vi "niRFSysCalReader Core.vi"(4 "Enable Interpolation?":bool=TRUE, 6 "CalData":dbl[](array[numeric]), 7 "Frequency (Hz)":dbl, 8 "error in":errorcluster, 9 "niRFSysCalReader State":T1, 10 "Power (dBm)":dbl, 11 "niRFSysCalReader Handle":T2) -> (0 "error out":errorcluster, 2 "CalData Out":dbl[](array[numeric]), 3 "niRFSysCalReader Handle out":T2)   [LabVIEW 2018, in "niRFSysCalReader.lvlib"]
doc: "Core component of the niRFSysCalReader library."
uses:
  niRFSysCalReader.lvlib
  INCLUDES/niRFSysCalReader Handle.ctl
  INCLUDES/niRFSysCalReader Core States.ctl
  <vilib>/Utility/error.llb/Error Cluster From Error Code.vi
  <vilib>/ErrorRing/Error Ring.xnode
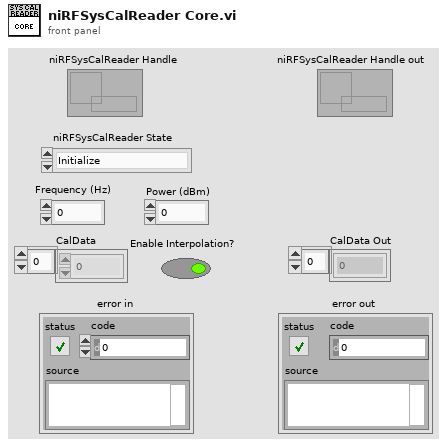
[diagram p1: front panel]
types:
  T1 = typedef "niRFSysCalReader.lvlib/niRFSysCalReader Core States.ctl" = enum16{"Initialize", "Interpolator State", "Add CalData", "Get CalData", "Remove Pathloss", "Close"}
  T2 = typedef "niRFSysCalReader.lvlib/niRFSysCalReader Handle.ctl" = refnum<data-value>
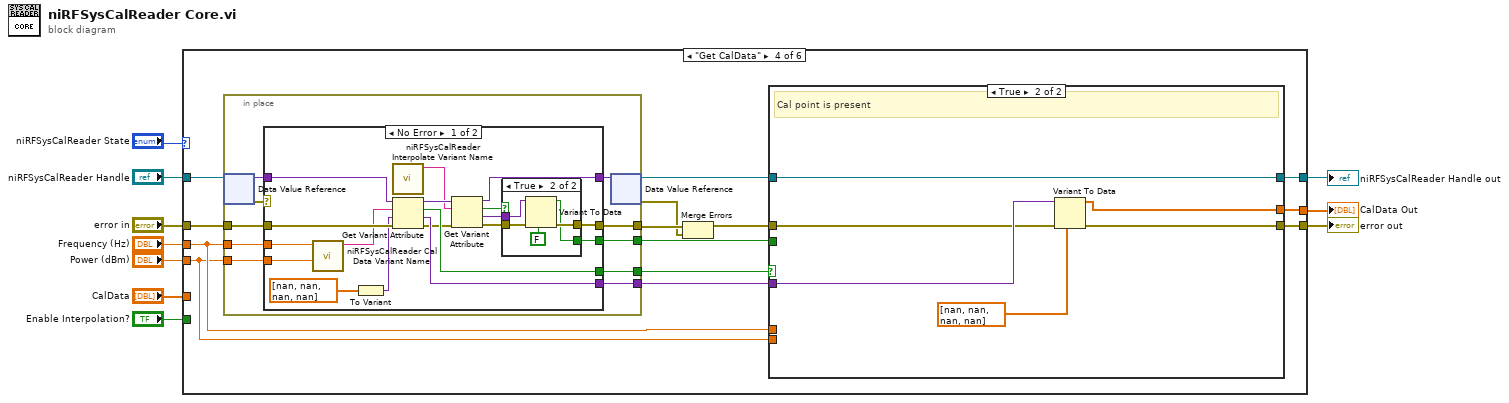
[diagram p0: block diagram]
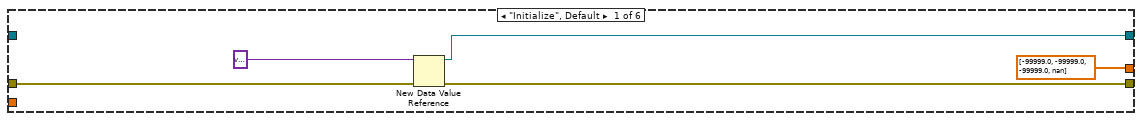
[diagram p2: hidden frame]
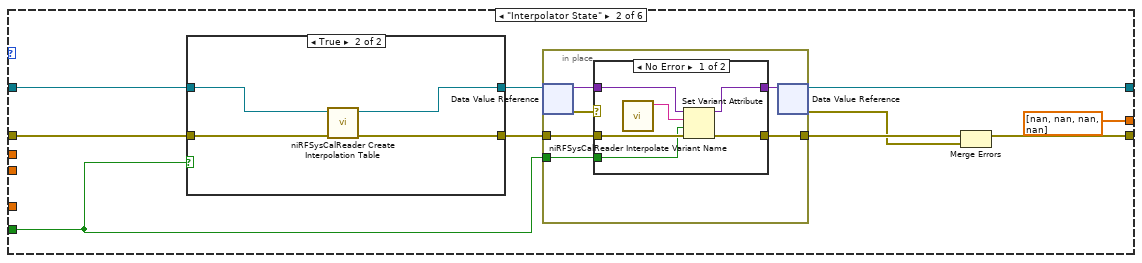
[diagram p3: hidden frame]
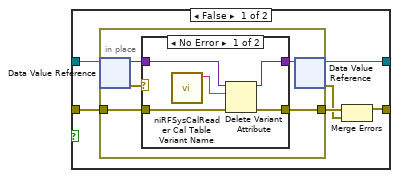
[diagram p4: hidden frame]
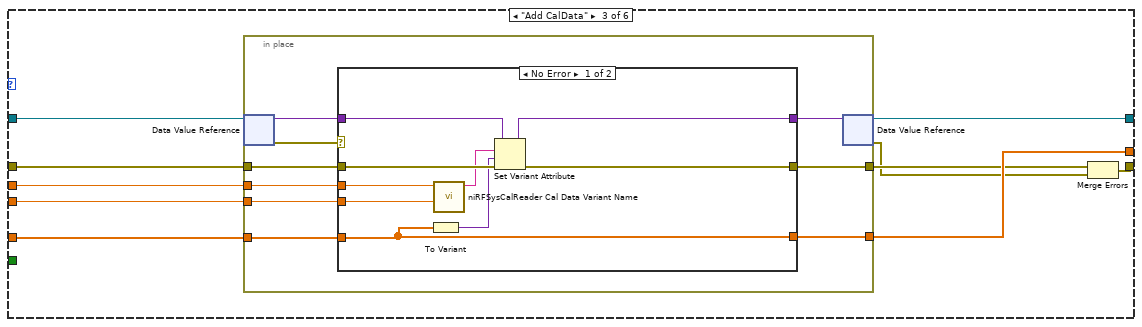
[diagram p7: hidden frame]
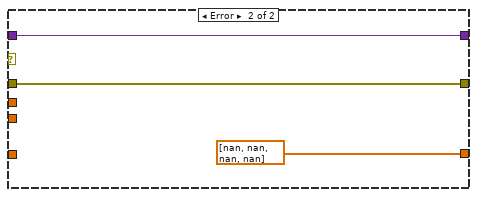
[diagram p8: hidden frame]
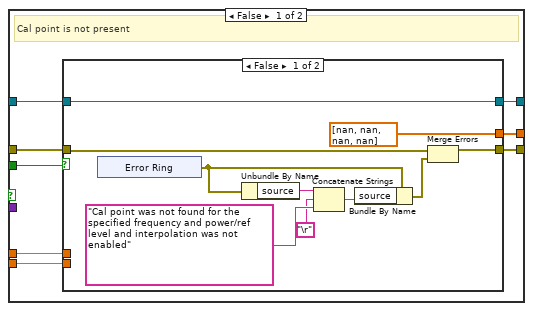
[diagram p9: hidden frame]
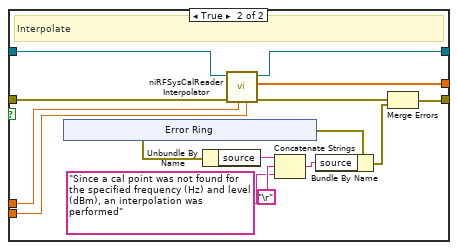
[diagram p10: hidden frame]
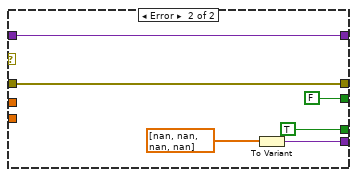
[diagram p12: hidden frame]
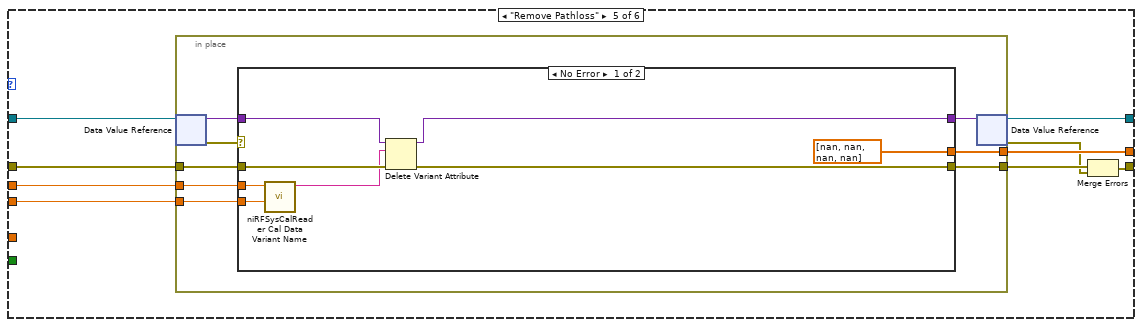
[diagram p13: hidden frame]
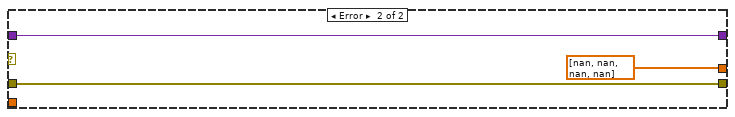
[diagram p14: hidden frame]
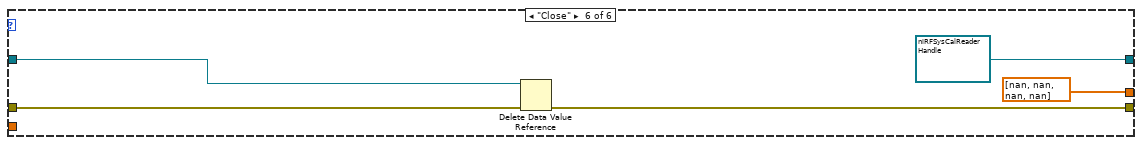
[diagram p15: hidden frame]
diagram:
  n1 = case shown="\"Get CalData\"" "niRFSysCalReader State" {
    tunnel: [w14 w25 w69 w97 w200 T2 refnum ("Cal Storage Handle in")] -> w5
    tunnel: [w13 w24 w68 w100 w199 w224] -> w4
    tunnel: "error in" -> [w12 w21 w70 w105 w201 w225]
    tunnel: "niRFSysCalReader Handle" -> [_ w23 w71 w106 w202 w226]
    tunnel: "Frequency (Hz)" -> [_ _ w67 w96 w198 _]
    tunnel: "Power (dBm)" -> [_ _ w66 w95 w197 _]
    tunnel: [dbl[] [-99999.0, -99999.0, -99999.0, nan] dbl[] [nan, nan, nan, nan] w65 w99 w196 dbl[] [nan, nan, nan, nan]] -> w1
    tunnel: "Enable Interpolation?" -> [_ w17 _ _ _ _]
    tunnel: "CalData" -> [_ _ w62 _ _ _]
    frame "Initialize", Default {
      n2 = New Data Value Reference(data value=variant, error in=w12) -> (data value reference=w14:refnum<data-value>, error out=w13:errorcluster)
    }
    frame "Interpolator State" {
      n3 = case shown="True" w17 {
        tunnel: w23 -> [w31 w47]
        tunnel: [w30 w46] -> w22
        tunnel: w21 -> [w29 w45]
        tunnel: [w28 w44] -> w20
        frame False {
          n4 = in-place {
            in-place-border: w29 -> [w34]
            in-place-border: [w33] -> w27
            n5 = in-place-dvr #1(w31) -> (w36:variant, w32:errorcluster)
            n6 = case shown="No Error" w32 {
              tunnel: w36 -> [w41 w43]
              tunnel: [w40 w43] -> w35
              tunnel: w34 -> [w39 w42]
              tunnel: [w38 w42] -> w33
              frame No Error {
                n7 = call "niRFSysCalReader Cal Table Variant Name.vi"() -> ("Calibration Table Name"=w37:string)  [unwired: 11 in]
                n8 = Delete Variant Attribute(4:w39, 6:w37, 7:w41) -> (0:w38:errorcluster, 3:w40:variant)  [unwired: 1 out]
              }
              frame Error {
              }
            }
            n9 = in-place-dvr #1(w35) -> (w30:T2, w26:errorcluster)
          }
          n10 = Merge Errors(w27, w26) -> (w28:errorcluster)
        }
        frame True {
          n11 = call "niRFSysCalReader Create Interpolation Table.vi"("error in"=w45, "niRFSysCalReader Handle"=w47) -> ("error out"=w44:errorcluster, "niRFSysCalReader Handle out"=w46:T2)  [unwired: 7 in, 1 out]
        }
      }
      n12 = in-place {
        in-place-border: [w52] -> w19
        in-place-border: w20 -> [w50]
        in-place-border: w17 -> [w48]
        n13 = in-place-dvr #2(w22) -> (w53:variant, w49:errorcluster)
        n14 = case shown="No Error" w49 {
          tunnel: w53 -> [w59 w61]
          tunnel: [w57 w60] -> w52
          tunnel: [w56 w61] -> w51
          tunnel: w50 -> [w55 w60]
          tunnel: w48 -> [w54 _]
          frame No Error {
            n15 = call "niRFSysCalReader Interpolate Variant Name.vi"() -> ("Interpolation State Name"=w58:string)  [unwired: 11 in]
            n16 = Set Variant Attribute(Variant=w59, name=w58, value=w54, error in=w55) -> (Variant out=w56:variant, error out=w57:errorcluster)  [unwired: 1 out]
          }
          frame Error {
          }
        }
        n17 = in-place-dvr #2(w51) -> (w25:T2, w18:errorcluster)
      }
      n18 = Merge Errors(w19, w18) -> (w24:errorcluster)
    }
    frame "Add CalData" {
      n19 = in-place {
        in-place-border: w70 -> [w79]
        in-place-border: [w76] -> w64
        in-place-border: w67 -> [w75]
        in-place-border: w66 -> [w74]
        in-place-border: [w73] -> w65
        in-place-border: w62 -> [w72]
        n20 = in-place-dvr #3(w71) -> (w78:variant, w80:errorcluster)
        n21 = case shown="No Error" w80 {
          tunnel: w79 -> [w89 w91]
          tunnel: w78 -> [w84 w92]
          tunnel: [w83 w92] -> w77
          tunnel: [w88 w91] -> w76
          tunnel: w75 -> [w87 _]
          tunnel: w74 -> [w86 _]
          tunnel: w72 -> [w81 _]
          tunnel: [w81 dbl[] [nan, nan, nan, nan]] -> w73
          frame No Error {
            n22 = To Variant(anything=w81) -> (Variant=w82:variant)
            n23 = call "niRFSysCalReader Cal Data Variant Name.vi"("Power (dBm)"=w86, "Frequency (Hz)"=w87) -> ("Calibration Data Name"=w85:string)  [unwired: 9 in]
            n24 = Set Variant Attribute(Variant=w84, name=w85, value=w82, error in=w89) -> (Variant out=w83:variant, error out=w88:errorcluster)  [unwired: 1 out]
          }
          frame Error {
          }
        }
        n25 = in-place-dvr #3(w77) -> (w69:T2, w63:errorcluster)
      }
      n26 = Merge Errors(w64, w63) -> (w68:errorcluster)
    }
    frame "Get CalData" {
      n27 = in-place {
        in-place-border: w105 -> [w161]
        in-place-border: [w158] -> w104
        in-place-border: w96 -> [w157]
        in-place-border: w95 -> [w156]
        in-place-border: [w155] -> w93
        in-place-border: [w154] -> w102
        in-place-border: [w153] -> w94
        n28 = in-place-dvr #4(w106) -> (w160:variant, w162:errorcluster)
        n29 = case shown="No Error" w162 {
          tunnel: w161 -> [w180 w192]
          tunnel: w160 -> [w178 w193]
          tunnel: [w170 w193] -> w159
          tunnel: [w168 w192] -> w158
          tunnel: w157 -> [w176 _]
          tunnel: w156 -> [w175 _]
          tunnel: [w174 w188] -> w154
          tunnel: [w173 TRUE] -> w155
          tunnel: [w165 FALSE] -> w153
          frame No Error {
            n30 = call "niRFSysCalReader Cal Data Variant Name.vi"("Power (dBm)"=w175, "Frequency (Hz)"=w176) -> ("Calibration Data Name"=w179:string)  [unwired: 9 in]
            n31 = To Variant(anything=dbl[] [nan, nan, nan, nan]) -> (Variant=w177:variant)
            n32 = call "niRFSysCalReader Interpolate Variant Name.vi"() -> ("Interpolation State Name"=w164:string)  [unwired: 11 in]
            n33 = Get Variant Attribute(Variant=w178, name=w179, default value (empty Variant)=w177, error in=w180) -> (duplicate Variant=w171:variant, found=w173:bool, value=w174:variant, error out=w172:errorcluster)
            n34 = Get Variant Attribute(Variant=w171, name=w164, error in=w172) -> (duplicate Variant=w170:variant, found=w166:bool, value=w167:variant, error out=w169:errorcluster)  [unwired: 1 in]
            n35 = case shown="True" w166 {
              selector: w166 -> [w182 _]
              tunnel: w169 -> [w181 w187]
              tunnel: [w181 w186] -> w168
              tunnel: w167 -> [_ w185]
              tunnel: [w182 w183] -> w165
              frame False {
              }
              frame True {
                n36 = Variant To Data(error in=w187, type=FALSE, Variant=w185) -> (data=w183:bool, error out=w186:errorcluster)
              }
            }
          }
          frame Error {
            n37 = To Variant(anything=dbl[] [nan, nan, nan, nan]) -> (Variant=w188:variant)
          }
        }
        n38 = in-place-dvr #4(w159) -> (w98:T2, w103:errorcluster)
      }
      n39 = Merge Errors(w104, w103) -> (w101:errorcluster)
      n40 = case shown="True" w93 {
        tunnel: [w114 w152] -> w100
        tunnel: [w113 w151] -> w99
        tunnel: w102 -> [_ w150]
        tunnel: w101 -> [w112 w149]
        tunnel: w98 -> [w111 w148]
        tunnel: [w110 w148] -> w97
        tunnel: w94 -> [w109 _]
        tunnel: w96 -> [w108 _]
        tunnel: w95 -> [w107 _]
        frame False {
          # "Cal point is not present"
          n41 = case shown="False" w109 {
            tunnel: [w122 w134] -> w114
            tunnel: [dbl[] [nan, nan, nan, nan] w142] -> w113
            tunnel: w112 -> [w123 w141]
            tunnel: w111 -> [w124 w140]
            tunnel: [w124 w139] -> w110
            tunnel: w108 -> [_ w130]
            tunnel: w107 -> [_ w129]
            frame False {
              n42 = xnode "Error Ring"() -> ("error out"=w121:errorcluster)
              n43 = Unbundle By Name(w121) -> ("source"=w118:string)
              n44 = Concatenate Strings(w118, "\r", "Cal point was not found for the specified frequency and power/ref level and interpolation was not enabled" ("error message (\"\")")) -> (w117:string)
              n45 = Bundle By Name(cluster=w121, "source"=w117) -> (w116:errorcluster)
              n46 = Merge Errors(w123, w116) -> (w122:errorcluster)
            }
            frame True {
              # "Interpolate"
              n47 = xnode "Error Ring"() -> ("error out"=w131:errorcluster)
              n48 = Unbundle By Name(w131) -> ("source"=w137:string)
              n49 = call "niRFSysCalReader Interpolator.vi"("Power (dBm)"=w129, "Frequency (Hz)"=w130, "error in"=w141, "niRFSysCalReader Handle"=w140) -> ("error out"=w133:errorcluster, "Interpolated Pathloss (dB)"=w142:dbl[], "niRFSysCalReader Handle out"=w139:T2)  [unwired: 5 in]
              n50 = Concatenate Strings(w137, "\r", "Since a cal point was not found for the specified frequency (Hz) and level (dBm), an interpolation was performed" ("error message (\"\")")) -> (w138:string)
              n51 = Bundle By Name(cluster=w131, "source"=w138) -> (w132:errorcluster)
              n52 = Merge Errors(w133, w132) -> (w134:errorcluster)
            }
          }
        }
        frame True {
          # "Cal point is present"
          n53 = Variant To Data(error in=w149, type=dbl[] [nan, nan, nan, nan], Variant=w150) -> (data=w151:dbl[], error out=w152:errorcluster)
        }
      }
    }
    frame "Remove Pathloss" {
      n54 = in-place {
        in-place-border: w201 -> [w209]
        in-place-border: [w206] -> w195
        in-place-border: w198 -> [w205]
        in-place-border: w197 -> [w204]
        in-place-border: [w203] -> w196
        n55 = in-place-dvr #5(w202) -> (w208:variant, w210:errorcluster)
        n56 = case shown="No Error" w210 {
          tunnel: w209 -> [w218 w220]
          tunnel: w208 -> [w214 w221]
          tunnel: [w213 w221] -> w207
          tunnel: [w215 w220] -> w206
          tunnel: w205 -> [w217 _]
          tunnel: w204 -> [w216 _]
          tunnel: [dbl[] [nan, nan, nan, nan] dbl[] [nan, nan, nan, nan]] -> w203
          frame No Error {
            n57 = call "niRFSysCalReader Cal Data Variant Name.vi"("Power (dBm)"=w216, "Frequency (Hz)"=w217) -> ("Calibration Data Name"=w212:string)  [unwired: 9 in]
            n58 = Delete Variant Attribute(4:w218, 6:w212, 7:w214) -> (0:w215:errorcluster, 3:w213:variant)  [unwired: 1 out]
          }
          frame Error {
          }
        }
        n59 = in-place-dvr #5(w207) -> (w200:T2, w194:errorcluster)
      }
      n60 = Merge Errors(w195, w194) -> (w199:errorcluster)
    }
    frame "Close" {
      n61 = Delete Data Value Reference(data value reference=w226, error in=w225) -> (error out=w224:errorcluster)  [unwired: 1 out]
    }
  }
  "niRFSysCalReader Handle out" <- w5
  "error out" <- w4
  "CalData Out" <- w1
